vi "SS measure.vi"(6 "AC sync source":T2, 7 "Common properties":T4={"Measurement status ref"=refnum, "TWM Status ref"=refnum, "Abort ref"=refnum, "Skip waiting ref"=refnum, "GNU Octave path"=path "C:/Program Files/GNU Octave/Octave-6.2.0/mingw64/bin", "TWM+QWTB path"=path "C:/Users/labina/Desktop/TWM-1.8.7.0-full/octprog", "lvlib path"=path "D:/martin/WAC/WACsw - github/control_software/Filter function meter/external libraries/GOLPI 0.7.3.1 source distribution LV 20.0 32 bit/lv_proc.dll", "TWM pipe"="\\\\.\\pipe\\TWM:server", "PJVS status ref"=refnum, "WAC path"=path ""}, 8 "error in (no error)":errorcluster, 9 "PJVS":T5={"PJVS type"=enum."AC-supraVOLTcontrol", "Status Refnum"=refnum, "AC-supraVOLTcontrol"={"IP address:port (0.0.0.0:0000)"="0.0.0.0:0000", "Timeouts"={"TCP Read & Write (ms)"=7000, "Sensors readout"=5000, "PJVS setup"=10000, "Nullmeter readout"=5000, "Multiplexer setup"=3000, "57XX setup"=15000, "Generator setup"=5000, "Synthesizer setup"=3000, "Sampler readout"=10000}, "Simulation mode"=FALSE, "Debug mode"=FALSE}, "NPL bias source"={"DataSocketCluster"={"Server Machine"="CZC105BD8M", "Client Machine"="localhost", "Data"="P2", "TimeStamp"=0.0, "Count"=1, "Target Process"="General Server"}}, "Manual PJVS"={"PJVS frequency (Hz)"=0.0, "Reference voltages (V)"=[], "File with PJVS voltages"=path ""}, "VTT PJVS"={"some VTT only property"=""}} {"NPL bias source"."DataSocketCluster"."TimeStamp" format="%.2f"}, 10 "AC Source":T2, 11 "SS measurement":T1={"Signal frequencies (Hz)"=[1000.0], "Signal amplitudes (V)"=[0.707], "Sampling frequencies (Hz)"=[10000000.0], "Record lengths (multiples of periods)"=[10000.0], "Calculate results"=FALSE, "Algorithm"="TWM-PJVSSubS", "TWM data directories"=[], "TWM data directories relative"=[], "Settle down after AC source change (s)"=1.0, "PJVS frequencies (Hz)"=[1000.0], "PJVS reference voltages array of vector cluster"=[{"PJVS reference voltages vector"=[]}], "Requested PJVS steps"=[20], "Measure CE"=FALSE, "Measure CE before"=FALSE, "Measure CE after"=FALSE, "Single point CE measurement"=FALSE, "original CE template path"=path "", "new CE template path before SS"=path "", "new CE template path before SS relative"=path "", "new CE template path after SS"=path "", "new CE template path after SS relative"=path "", "original CE fit path"=path "", "new CE fit path before SS"=path "", "new CE fit path before SS relative"=path "", "new CE fit path after SS"=path "", "new CE fit path after SS relative"=path "", "Measure digitizer gain"=FALSE, "Measure digitizer gain before"=FALSE, "Measure digitizer gain after"=FALSE, "Digitizer gain"=0.0, "Data folder"=path "", "FR fit path"=path "", "new FR fit path relative"=path "", "Rs"=0, "Re"=0, "SS measurement info files"=[]} {"PJVS reference voltages array of vector cluster"."PJVS reference voltages vector" format="%#_3p"; "PJVS frequencies (Hz)" format="%#_3p"; "Record lengths (multiples of periods)" format="%#_3p"; "Sampling frequencies (Hz)" format="%#_3p"; "Signal amplitudes (V)" format="%#_3p"; "Signal frequencies (Hz)" format="%#_3p"}) -> (0 "error out":errorcluster)   [LabVIEW 2020]
doc: "Runs a series of subsampling measurements."
uses:
  Type definitions/SS measurement.ctl
  General AC source/Type definitions/AC Source.ctl
  General AC source/Type definitions/AC Source type.ctl
  General PJVS driver/Type definitions/PJVS.ctl
  General PJVS driver/Type definitions/PJVS Type.ctl
  external libraries/acsvcontrol-driver/Public/Type Definitions/Timeouts.ctl
  external libraries/JV modified NPL Bias source/DataSocketCluster external.ctl
  Utilities/Type definitions/Common properties.ctl
  Utilities/Type definitions/Sampling properties.ctl
  <vilib>/Utility/error.llb/DialogType.ctl
  external libraries/TWM-1.8.7.0-client/TWM Client.lvlib
  external libraries/varilib/varilib.lvlib
  external libraries/acsvcontrol-driver/ACSVcontrol-driver.lvlib
panel:
  out "SS measurement out":T1={"Signal frequencies (Hz)"=[1000.0], "Signal amplitudes (V)"=[0.707], "Sampling frequencies (Hz)"=[10000000.0], "Record lengths (multiples of periods)"=[10000.0], "Calculate results"=FALSE, "Algorithm"="TWM-PJVSSubS", "TWM data directories"=[], "TWM data directories relative"=[], "Settle down after AC source change (s)"=1.0, "PJVS frequencies (Hz)"=[1000.0], "PJVS reference voltages array of vector cluster"=[{"PJVS reference voltages vector"=[]}], "Requested PJVS steps"=[20], "Measure CE"=FALSE, "Measure CE before"=FALSE, "Measure CE after"=FALSE, "Single point CE measurement"=FALSE, "original CE template path"=path "", "new CE template path before SS"=path "", "new CE template path before SS relative"=path "", "new CE template path after SS"=path "", "new CE template path after SS relative"=path "", "original CE fit path"=path "", "new CE fit path before SS"=path "", "new CE fit path before SS relative"=path "", "new CE fit path after SS"=path "", "new CE fit path after SS relative"=path "", "Measure digitizer gain"=FALSE, "Measure digitizer gain before"=FALSE, "Measure digitizer gain after"=FALSE, "Digitizer gain"=0.0, "Data folder"=path "", "FR fit path"=path "", "new FR fit path relative"=path "", "Rs"=0, "Re"=0, "SS measurement info files"=[]} {"PJVS reference voltages array of vector cluster"."PJVS reference voltages vector" format="%#_3p"; "PJVS frequencies (Hz)" format="%#_3p"; "Record lengths (multiples of periods)" format="%#_3p"; "Sampling frequencies (Hz)" format="%#_3p"; "Signal amplitudes (V)" format="%#_3p"; "Signal frequencies (Hz)" format="%#_3p"}
  out "TWM handle":i32
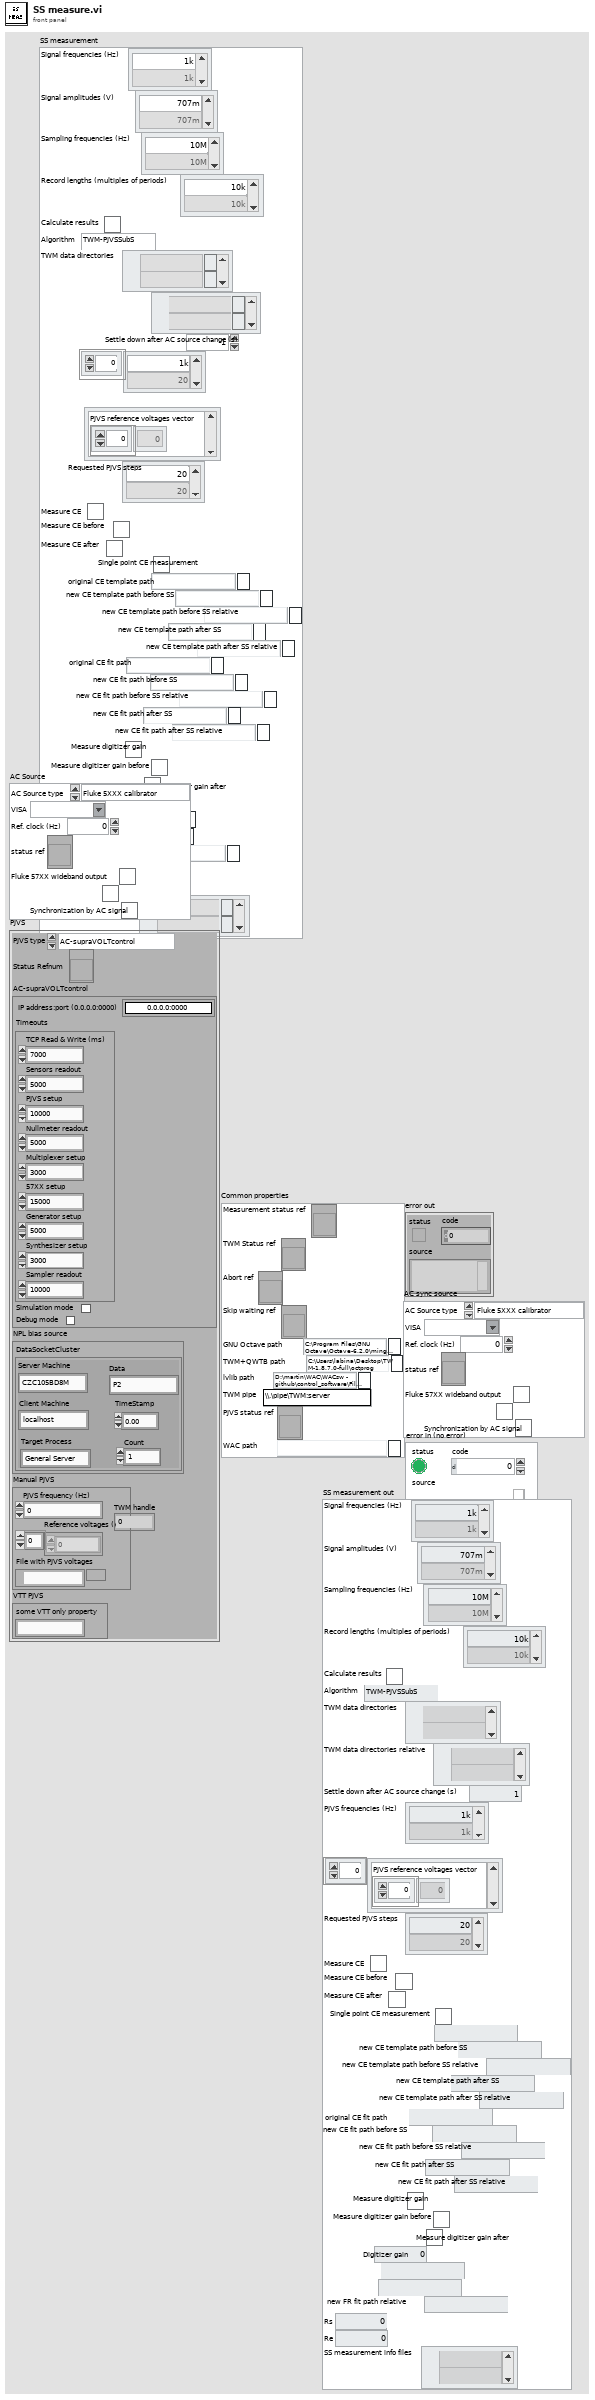
[diagram p1: front panel]
types:
  T1 = typedef "SS measurement.ctl" = cluster{"Signal frequencies (Hz)":dbl[], "Signal amplitudes (V)":dbl[], "Sampling frequencies (Hz)":dbl[], "Record lengths (multiples of periods)":dbl[], "Calculate results":bool, "Algorithm":string, "TWM data directories":path[], "TWM data directories relative":path[], "Settle down after AC source change (s)":dbl, "PJVS frequencies (Hz)":dbl[], "PJVS reference voltages array of vector cluster":cluster{"PJVS reference voltages vector":dbl[]}[], "Requested PJVS steps":u32[], "Measure CE":bool, "Measure CE before":bool, "Measure CE after":bool, "Single point CE measurement":bool, "original CE template path":path, "new CE template path before SS":path, "new CE template path before SS relative":path, "new CE template path after SS":path, "new CE template path after SS relative":path, "original CE fit path":path, "new CE fit path before SS":path, "new CE fit path before SS relative":path, "new CE fit path after SS":path, "new CE fit path after SS relative":path, "Measure digitizer gain":bool, "Measure digitizer gain before":bool, "Measure digitizer gain after":bool, "Digitizer gain":dbl, "Data folder":path, "FR fit path":path, "new FR fit path relative":path, "Rs":i32, "Re":i32, "SS measurement info files":path[]}
  T2 = typedef "AC Source.ctl" = cluster{"AC Source type":T3, "VISA":refnum<visa-resource-name>, "Ref. clock (Hz)":dbl, "status ref":refnum<vi>, "Fluke 57XX wideband output":bool, "Fluke 57XX ignore errors":bool, "Synchronization by AC signal":bool}
  T3 = typedef "AC Source type.ctl" = enum16{"Fluke 5XXX calibrator", "Tektronix AFG3000 series", "dummy", "Agilent 331xxA to 332xxA", "Agilent 335xxA to 336xxA"}
  T4 = typedef "Common properties.ctl" = cluster{"Measurement status ref":refnum<vi>, "TWM Status ref":refnum<vi>, "Abort ref":refnum<vi>, "Skip waiting ref":refnum<vi>, "GNU Octave path":path, "TWM+QWTB path":path, "lvlib path":path, "TWM pipe":string, "PJVS status ref":refnum<vi>, "WAC path":path}
  T5 = typedef "PJVS.ctl" = cluster{"PJVS type":T6, "Status Refnum":refnum<vi>, "AC-supraVOLTcontrol":cluster{"IP address:port (0.0.0.0:0000)":string, "Timeouts":T7, "Simulation mode":bool, "Debug mode":bool}, "NPL bias source":cluster{"DataSocketCluster":T8}, "Manual PJVS":cluster{"PJVS frequency (Hz)":dbl, "Reference voltages (V)":dbl[], "File with PJVS voltages":path}, "VTT PJVS":cluster{"some VTT only property":string}}
  T6 = typedef "PJVS Type.ctl" = enum16{"AC-supraVOLTcontrol", "JV modified NPL bias control", "Manual PJVS", "VTT PJVS"}
  T7 = typedef "ACSVcontrol-driver.lvlib/Timeouts.ctl" = cluster{"TCP Read & Write (ms)":i32, "Sensors readout":i32, "PJVS setup":i32, "Nullmeter readout":i32, "Multiplexer setup":i32, "57XX setup":i32, "Generator setup":i32, "Synthesizer setup":i32, "Sampler readout":i32}
  T8 = typedef "DataSocketCluster external.ctl" = cluster{"Server Machine":string, "Client Machine":string, "Data":string, "TimeStamp":dbl, "Count":i32, "Target Process":string}
  T9 = typedef "Sampling properties.ctl" = cluster{"Sampling frequency (Hz)":dbl, "Record length (multiples of period)":dbl, "Signal amplitude (V)":dbl, "Measurement frequency (Hz)":dbl, "Calculate RMS from samples":bool, "Algorithm":string, "Measurement path":string}
  T10 = cluster{"PJVS reference voltages vector":dbl[]}[]
  T11 = typedef "DialogType.ctl" = u16
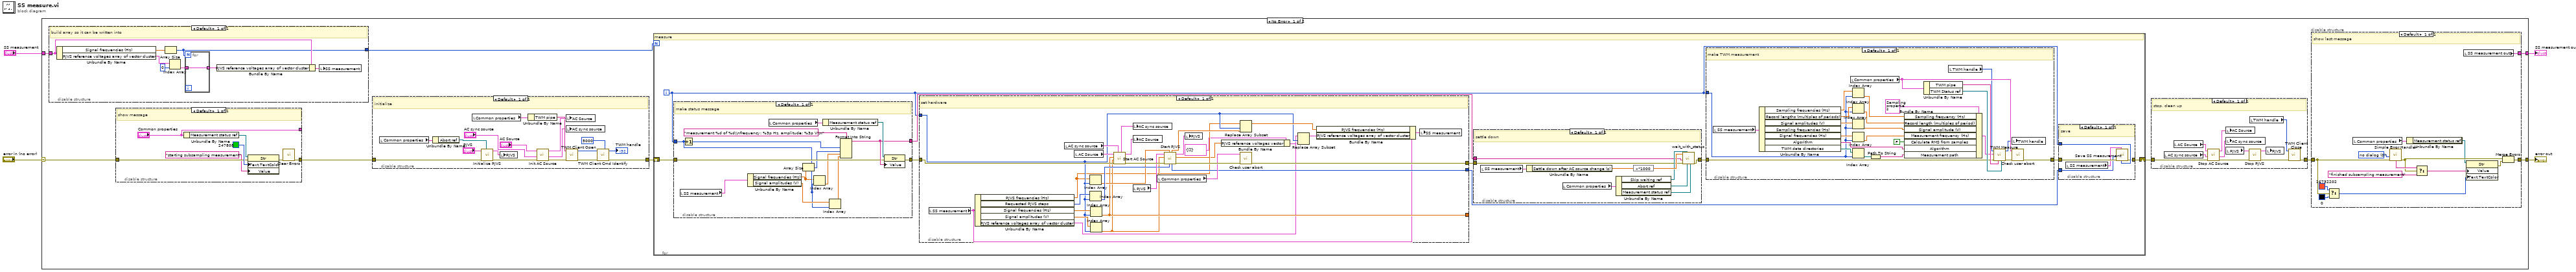
[diagram p0: block diagram]
diagram:
  n1 = case shown="No Error" "error in (no error)" {
    selector: "error in (no error)" -> [w8 w167]
    tunnel: [w13 w167] -> w4
    tunnel: "SS measurement" -> [w6 w166]
    tunnel: [w7 w166] -> w1
    frame No Error {
      n2 = disable-structure shown="Default" {
        disable-tunnel: w6 -> [w20]
        disable-tunnel: [w19] -> w5
        frame Enabled {
          # "build array so it can be written into"
          n3 = Unbundle By Name(w20) -> ("Signal frequencies (Hz)"=w21:dbl[], "PJVS reference voltages array of vector cluster"=w18:T10)
          n4 = Array Size(array=w21) -> (size(s)=w19:i32)
          n5 = Index Array(array=w18, index=0) -> (element=w17:cluster{"PJVS reference voltages vector":dbl[]})
          n6 = for {
            N: w19 -> [_]
            tunnel: w17 -> [w22]
            tunnel: [w22] -> w16 mode=indexing
          }
          n7 = Bundle By Name(cluster=w20, "PJVS reference voltages array of vector cluster"=w16) -> (w14:T1)
          n8 = local write "SS measurement"(w14) -> ()
        }
      }
      n9 = disable-structure shown="Default" {
        disable-tunnel: w8 -> [w163]
        disable-tunnel: ["Common properties"] -> _
        disable-tunnel: [w159] -> w12
        frame Enabled {
          # "show message"
          n10 = Unbundle By Name("Common properties") -> ("Measurement status ref"=w161:refnum<vi>)
          n11 = property class="Str"(reference=w161, error in=w163, "Text.TextColor"=u32 247808 ("Text.Text Colors:Text Color"), "Value"="starting subsampling measurement") -> (error out=w164:errorcluster)  [unwired: 1 out]
          n12 = call <vilib>:"Clear Errors.vi"("error in (no error)"=w164) -> ("error out"=w159:errorcluster)  [unwired: 5 in, 1 out]
        }
      }
      n13 = disable-structure shown="Default" {
        disable-tunnel: w12 -> [w137]
        disable-tunnel: [w129] -> w11
        frame Enabled {
          # "initialize"
          n14 = local read "Common properties"() -> (w142:T4)
          n15 = Unbundle By Name(w142) -> ("Abort ref"=w141:refnum<vi>)
          n16 = local read "Common properties"() -> (w131:T4)
          n17 = call "Initialize PJVS.vi"("Abort Refnum"=w141, "error in (no error)"=w137, "PJVS setup"="PJVS") -> ("error out"=w144:errorcluster, "PJVS setup out"=w140:T5)  [unwired: 7 in]
          n18 = local write "PJVS"(w140) -> ()
          n19 = Unbundle By Name(w131) -> ("TWM pipe"=w132:string)
          n20 = call "Init AC Source.vi"("error in (no error)"=w144, "AC sync source"="AC sync source", "AC source"="AC Source") -> ("error out"=w130:errorcluster, "AC sync source out"=w127:T2, "AC source out"=w138:T2)  [unwired: 5 in, 1 out]
          n21 = local write "AC Source"(w138) -> ()
          n22 = local write "AC sync source"(w127) -> ()
          n23 = call "TWM Client Open.vi"("error in"=w130, "pipe name"=w132) -> ("error out"=w135:errorcluster, "handle out"=w136:i32)  [unwired: 8 in]
          n24 = call "TWM Client Cmd Identify.vi"("timeout [ms]"=5000, "error in"=w135, "handle"=w136) -> ("error out"=w129:errorcluster, "handle out"=→"TWM handle":i32)  [unwired: 5 in, 2 out]
        }
      }
      n25 = for {
        N: w5 -> [_]
        shift-right: [w26] -> w10
        shift-left: w11 -> [w30]
        i -> [w23]
        # "measure"
        n26 = disable-structure shown="Default" {
          disable-tunnel: w23 -> [w94]
          disable-tunnel: [w101] -> w31
          disable-tunnel: w30 -> [w100]
          disable-tunnel: [w99] -> w29
          frame Enabled {
            # "make status message"
            n27 = local read "SS measurement"() -> (w98:T1)
            n28 = Increment(x=w94) -> (x+1=w102:i32)
            n29 = Unbundle By Name(w98) -> ("Signal frequencies (Hz)"=w93:dbl[], "Signal amplitudes (V)"=w97:dbl[])
            n30 = local read "Common properties"() -> (w104:T4)
            n31 = Array Size(array=w93) -> (size(s)=w92:i32)
            n32 = Index Array(array=w93, index=w94) -> (element=w95:dbl)
            n33 = Unbundle By Name(w104) -> ("Measurement status ref"=w105:refnum<vi>)
            n34 = Index Array(array=w97, index=w94) -> (element=w96:dbl)
            n35 = Format Into String(format string="measurement %d of %d\\nfrequency: %3p Hz, amplitude: %3p V\\n", w102, w92, w95, w96) -> (resulting string=w101:string)  [unwired: 2 in, 1 out]
            n36 = property class="Str"(reference=w105, error in=w100, "Value"=w101) -> (error out=w99:errorcluster)  [unwired: 1 out]
          }
        }
        n37 = disable-structure shown="Default" {
          disable-tunnel: w29 -> [w86]
          disable-tunnel: [w84] -> w28
          disable-tunnel: [w80] -> w27
          disable-tunnel: [w71] -> _
          disable-tunnel: w23 -> [w68]
          frame Enabled {
            # "set hardware"
            n38 = local read "SS measurement"() -> (w67:T1)
            n39 = Unbundle By Name(w67) -> ("PJVS frequencies (Hz)"=w66:dbl[], "Requested PJVS steps"=w73:u32[], "Signal frequencies (Hz)"=w72:dbl[], "Signal amplitudes (V)"=w70:dbl[], "PJVS reference voltages array of vector cluster"=w65:T10)
            n40 = local read "AC sync source"() -> (w82:T2)
            n41 = local read "AC Source"() -> (w88:T2)
            n42 = Index Array(array=w66, index=w68) -> (element=w74:dbl)
            n43 = Index Array(array=w73, index=w68) -> (element=w75:u32)
            n44 = Index Array(array=w72, index=w68) -> (element=w71:dbl)
            n45 = Index Array(array=w70, index=w68) -> (element=w69:dbl)
            n46 = call "Start AC Source.vi"("AC sync source"=w82, "error in (no error)"=w86, "Signal amplitude (V)"=w69, "Signal frequency  (Hz)"=w71, "AC source"=w88) -> ("error out"=w91:errorcluster, "AC source out"=w87:T2, "AC sync source out"=w81:T2)  [unwired: 3 in, 1 out]
            n47 = local write "AC sync source"(w81) -> ()
            n48 = local write "AC Source"(w87) -> ()
            n49 = local read "PJVS"() -> (w90:T5)
            n50 = local read "Common properties"() -> (w83:T4)
            n51 = call "Start PJVS.vi"("Requiested PJVS steps"=w75, "Requested PJVS frequency (Hz)"=w74, "error in (pass through)"=w91, "Maximal signal amplitude (V)"=w69, "PJVS setup"=w90) -> ("error out"=w85:errorcluster, "PJVS reference voltages (1 period, V)"=w62:dbl[], "PJVS setup out"=w89:T5, "Set PJVS steps"=w80:u32, "Set frequency (Hz)"=w77:dbl)  [unwired: 2 in]
            n52 = local write "PJVS"(w89) -> ()
            n53 = Bundle By Name(cluster=cluster{"PJVS reference voltages vector":dbl[]} {"PJVS reference voltages vector"=[]} ("new element/subarray"), "PJVS reference voltages vector"=w62) -> (w63:cluster{"PJVS reference voltages vector":dbl[]})
            n54 = Replace Array Subset(array=w66, new element=w77, index=w68) -> (w76:dbl[])
            n55 = call "Check user abort.vi"("error in (no error)"=w85, "Common properties"=w83) -> ("error out"=w84:errorcluster)  [unwired: 9 in]
            n56 = Replace Array Subset(array=w65, new element=w63, index=w68) -> (w79:T10)
            n57 = Bundle By Name(cluster=w67, "PJVS frequencies (Hz)"=w76, "PJVS reference voltages array of vector cluster"=w79) -> (w78:T1)
            n58 = local write "SS measurement"(w78) -> ()
          }
        }
        n59 = disable-structure shown="Default" {
          disable-tunnel: w31 -> [w108]
          disable-tunnel: w28 -> [w107]
          disable-tunnel: [w106] -> w25
          frame Enabled {
            # "settle down"
            n60 = local read "SS measurement"() -> (w109:T1)
            n61 = Unbundle By Name(w109) -> ("Settle down after AC source change (s)"=w114:dbl)
            n62 = local read "Common properties"() -> (w110:T4)
            n63 = Unbundle By Name(w110) -> ("Skip waiting ref"=w113:refnum<vi>, "Abort ref"=w112:refnum<vi>, "Measurement status ref"=w111:refnum<vi>)
            n64 = expression code="x*1000"(w114) -> (w115:dbl)
            n65 = call "wait_with_status.vi"("stat ref"=w111, "stop ref"=w112, "second stop ref"=w113, "error in"=w107, "comment"=w108, "ms to wait"=w115) -> ("error out"=w106:errorcluster)  [unwired: 4 in, 1 out]
          }
        }
        n66 = disable-structure shown="Default" {
          disable-tunnel: w23 -> [w47]
          disable-tunnel: w25 -> [w38]
          disable-tunnel: [w37] -> w24
          frame Enabled {
            # "make TWM measurement"
            n67 = local read "SS measurement"() -> (w54:T1)
            n68 = Unbundle By Name(w54) -> ("Sampling frequencies (Hz)"=w58:dbl[], "Record lengths (multiples of periods)"=w56:dbl[], "Signal amplitudes (V)"=w53:dbl[], "Signal frequencies (Hz)"=w51:dbl[], "Algorithm"=w49:string, "TWM data directories"=w48:path[])  [unwired: 1 out]
            n69 = local read "Common properties"() -> (w44:T4)
            n70 = Index Array(array=w58, index=w47) -> (element=w57:dbl)
            n71 = Index Array(array=w56, index=w47) -> (element=w55:dbl)
            n72 = Index Array(array=w53, index=w47) -> (element=w52:dbl)
            n73 = Index Array(array=w51, index=w47) -> (element=w50:dbl)
            n74 = Index Array(array=w48, index=w47) -> (element=w46:path)
            n75 = Path To String(path=w46) -> (string=w59:string)
            n76 = Bundle By Name(cluster=T9 {"Sampling frequency (Hz)"=500000.0, "Record length (multiples of period)"=1000.0, "Signal amplitude (V)"=4.5, "Measurement frequency (Hz)"=1000.0, "Calculate RMS from samples"=FALSE, "Algorithm"="TWM-WFFT", "Measurement path"=""} ("TWM Measurement properties"), "Sampling frequency (Hz)"=w57, "Record length (multiples of period)"=w55, "Signal amplitude (V)"=w52, "Measurement frequency (Hz)"=w50, "Calculate RMS from samples"=FALSE, "Algorithm"=w49, "Measurement path"=w59) -> (w39:T9)
            n77 = Unbundle By Name(w44) -> ("TWM pipe"=w42:string, "TWM Status ref"=w43:refnum<vi>)
            n78 = local read "TWM handle"() -> (w40:i32)
            n79 = call "TWM Measure.vi"("TWM Status ref"=w43, "TWM pipe"=w42, "error in (no error)"=w38, "TWM Measurement properties"=w39, "TWM handle"=w40) -> ("error out"=w45:errorcluster, "TWM handle out"=w41:i32)  [unwired: 3 in, 2 out]
            n80 = local write "TWM handle"(w41) -> ()
            n81 = call "Check user abort.vi"("error in (no error)"=w45, "Common properties"=w44) -> ("error out"=w37:errorcluster)  [unwired: 9 in]
          }
        }
        n82 = disable-structure shown="Default" {
          disable-tunnel: w27 -> [w35]
          disable-tunnel: [w32] -> w26
          disable-tunnel: w24 -> [w36]
          disable-tunnel: w23 -> [w33]
          frame Enabled {
            # "save"
            n83 = local read "SS measurement"() -> (w34:T1)
            n84 = call "Save SS measurement.vi"("Index"=w33, "SS measurement"=w34, "error in"=w36, "Set PJVS steps"=w35) -> ("error out"=w32:errorcluster)  [unwired: 7 in]
          }
        }
      }
      n85 = disable-structure shown="Default" {
        disable-tunnel: [w117] -> w9
        disable-tunnel: w10 -> [w121]
        frame Enabled {
          # "stop, clean up"
          n86 = local read "AC sync source"() -> (w120:T2)
          n87 = local read "AC Source"() -> (w122:T2)
          n88 = call "Stop AC Source.vi"("error in (no error)"=w121, "AC sync source"=w120, "AC source"=w122) -> ("error out"=w126:errorcluster, "AC sync source out"=w119:T2, "AC source out"=w123:T2)  [unwired: 6 in]
          n89 = local write "AC Source"(w123) -> ()
          n90 = local write "AC sync source"(w119) -> ()
          n91 = local read "PJVS"() -> (w125:T5)
          n92 = call "Stop PJVS.vi"("error in (pass through)"=w126, "PJVS setup"=w125) -> ("error out"=w118:errorcluster, "PJVS setup out"=w124:T5)  [unwired: 8 in]
          n93 = local read "TWM handle"() -> (w116:i32)
          n94 = local write "PJVS"(w124) -> ()
          n95 = call "TWM Client Close.vi"("error in"=w118, "handle in"=w116) -> ("error out"=w117:errorcluster)  [unwired: 9 in]
        }
      }
      n96 = disable-structure shown="Default" {
        disable-tunnel: [w147] -> w13
        disable-tunnel: w9 -> [w146]
        disable-tunnel: [w145] -> w7
        frame Enabled {
          w155 = T11 0 items=["no dialog", "OK message", "continue or stop message", "OK message + warnings", "continue/stop + warnings"] ("type of dialog (OK msg:1)")
          # "show last message"
          n97 = Select(t=u32 16732202 ("Text.Text Colors:Text Color"), s=w146, f=u32 0 ("Text.Text Colors:Text Color")) -> (s? t:f=w152:u32)
          n98 = local read "Common properties"() -> (w148:T4)
          n99 = call <vilib>:"Simple Error Handler.vi"("type of dialog (OK msg:1)"=w155, "error in (no error)"=w146) -> ("error out"=w150:errorcluster, "message"=w158:string)  [unwired: 3 in, 3 out]
          n100 = Unbundle By Name(w148) -> ("Measurement status ref"=w149:refnum<vi>)
          n101 = Select(t=w158, s=w150, f="finished subsampling measurement") -> (s? t:f=w156:string)
          n102 = local read "SS measurement out"() -> (w145:T1)
          n103 = property class="Str"(reference=w149, "Value"=w156, "Text.TextColor"=w152) -> (error out=w151:errorcluster)  [unwired: 1 in, 1 out]
          n104 = Merge Errors(w150, w151) -> (w147:errorcluster)
        }
      }
    }
    frame Error {
    }
  }
  "error out" <- w4
  "SS measurement out" <- w1
